vi "update stim config control (sub-vi).vi"(7 "update ring entries? (T)":bool=TRUE, 8 "error in (no error)":errorcluster, 9 "changed? [] (empty)":bool[](array[boolean]), 10 "odor-manifold config":T1, 11 "stim. config array refnum":refnum<vi>) -> (0 "error out":errorcluster, 3 "stim. config array refnum out":refnum<vi>, 4 "value error":errorcluster)   [LabVIEW 2021]
uses:
  type-defs/odor and manifold config cluster (type def).ctl
  type-defs/manifold configuration cluster array (type def).ctl
  type-defs/manifold configuration cluster (type def).ctl
  type-defs/manifold selection.ctl
  type-defs/single port single odor cluster.ctl
  type-defs/port number (type def).ctl
  type-defs/odor selection (type def).ctl
  type-defs/odor color (type def).ctl
  type-defs/odor description array (type def).ctl
  type-defs/odor info cluster (type def).ctl
  type-defs/stimulation configuration array (type def).ctl
  type-defs/stimulator configuration line cluster (type def).ctl
  type-defs/port-odor with color cluster (type def).ctl
  type-defs/port-odor ring (type def).ctl
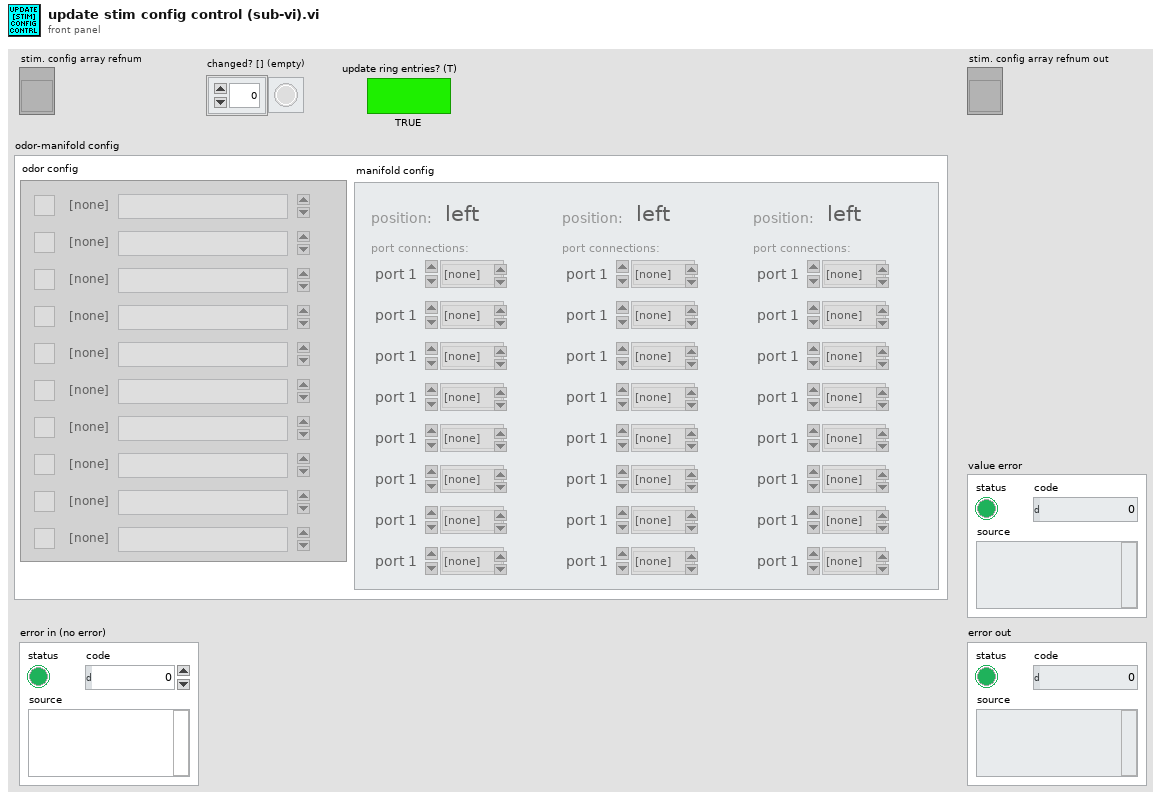
[diagram p1: front panel]
types:
  T1 = typedef "odor and manifold config cluster (type def).ctl" = cluster{"manifold config":T2, "odor config":T9}
  T2 = typedef "manifold configuration cluster array (type def).ctl" = T3[]
  T3 = typedef "manifold configuration cluster (type def).ctl" = cluster{"position:":T4, "port connections:":T5[]}
  T4 = typedef "manifold selection.ctl" = enum16{"left", "middle", "right"}
  T5 = typedef "single port single odor cluster.ctl" = cluster{"port number":T6, "connected odor":T7, "error":bool, "odor color":T8}
  T6 = typedef "port number (type def).ctl" = enum16{"port 1", "port 2", "port 3", "port 4", "port 5", "port 6", "port 7", "port 8"}
  T7 = typedef "odor selection (type def).ctl" = enum16{"[none]", "odor 1", "odor 2", "odor 3", "odor 4", "odor 5", "odor 6", "odor 7", "odor 8", "odor 9", "odor 10"}
  T8 = typedef "odor color (type def).ctl" = u16
  T9 = typedef "odor description array (type def).ctl" = T10[]
  T10 = typedef "odor info cluster (type def).ctl" = cluster{"odor channel":T7, "odor description":string, "odor color":T8, "odor channel active":bool}
  T11 = typedef "odor channel to odor color map (type def).ctl" = map{T7, T8}
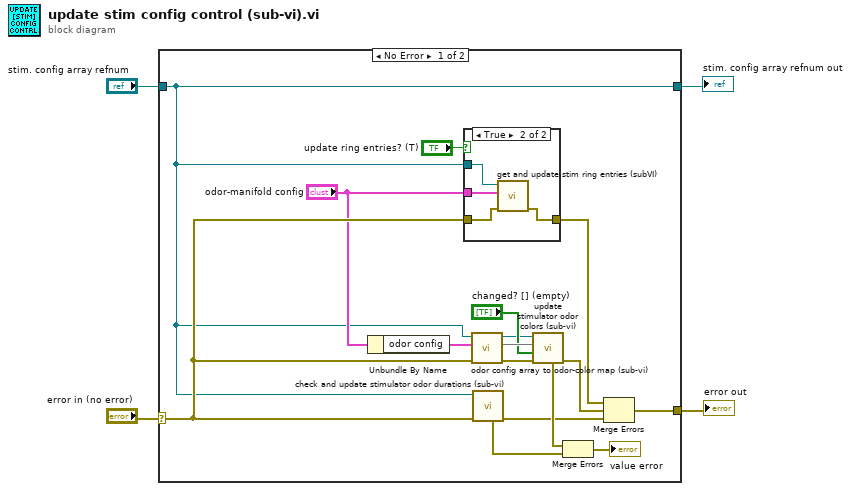
[diagram p0: block diagram]
diagram:
  n1 = case shown="No Error" "error in (no error)" {
    selector: "error in (no error)" -> [w10 w24]
    tunnel: [w15 w24] -> w3
    tunnel: "stim. config array refnum" -> [w4 w23]
    tunnel: [w4 w23] -> _
    frame No Error {
      n2 = Unbundle By Name("odor-manifold config") -> ("odor config"=w17:T9)
      n3 = case shown="True" "update ring entries? (T)" {
        tunnel: w10 -> [w18 w22]
        tunnel: "odor-manifold config" -> [_ w19]
        tunnel: [w18 w21] -> w7
        tunnel: w4 -> [_ w20]
        frame False {
        }
        frame True {
          n4 = call "get and update stim ring entries (subVI).vi"("error in (no error)"=w22, "odor-manifold config"=w19, "stim config array refnum"=w20) -> ("error out"=w21:errorcluster)  [unwired: 7 in, 1 out]
        }
      }
      n5 = call "odor config array to odor-color map (sub-vi).vi"("odor config array"=w17) -> ("odor-color map"=w16:T11)  [unwired: 10 in]
      n6 = call "check and update stimulator odor durations (sub-vi).vi"("error in (no error)"=w10, "stim. config array refnum"=w4) -> ("error out"=w5:errorcluster, "value error"=w13:errorcluster)  [unwired: 7 in, 1 out]
      n7 = call "update stimulator odor colors (sub-vi).vi"("error in (no error)"=w10, "changed? [] (empty, all true)"="changed? [] (empty)", "odor-color map"=w16, "stim. config array refnum"=w4) -> ("error out"=w6:errorcluster, "value error"=w8:errorcluster)  [unwired: 5 in, 1 out]
      n8 = Merge Errors(w8, w13) -> (→"value error":errorcluster)
      n9 = Merge Errors(w7, w6, w5) -> (w15:errorcluster)
    }
    frame Error {
    }
  }
  "error out" <- w3
  "stim. config array refnum out" <- "stim. config array refnum"
